vi "DAQmx Write (Raw 1D U32).vi"(0 "task/channels in":refnum<k21>, 1 "auto start":bool, 7 "data":u32[](array[numeric]), 9 "timeout":dbl=10.0 format="%0.2f", 11 "error in":errorcluster) -> (4 "task out":refnum<k21>, 10 "number of samples written per channel":u32, 15 "error out":errorcluster)   [LabVIEW 2022 SP3]
doc: "Writes multiple raw, 32-bit unsigned integer samples to a task. Use this instance for devices that use 32-bit unsigned integers as the internal representation of a sample."
uses:
  nilvaiu.dll
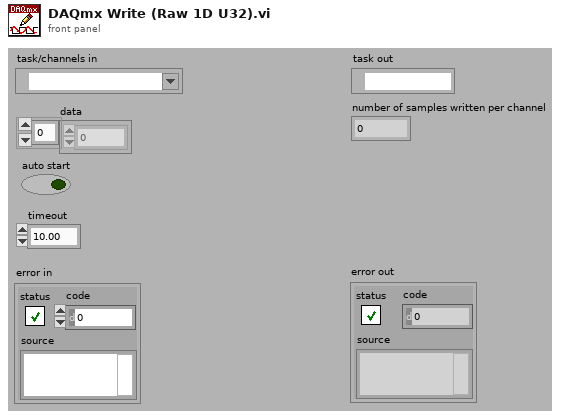
[diagram p1: front panel]
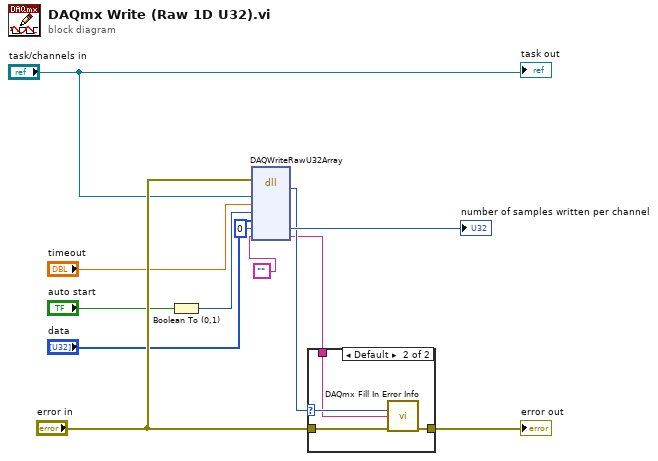
[diagram p0: block diagram]
diagram:
  n1 = Boolean To (0,1)(Boolean="auto start") -> (0, 1=w4:i16)
  n2 = dll-call lib="nilvaiu.*" fn="DAQWriteRawU32Array"(error in="error in", "taskID"="task/channels in", "timeout"="timeout", "autoStart"=w4, "data"="data", "numSamplesWriten"=u32 0, "extendedErrorInfo"="") -> ("return type"=w5:u32, "numSamplesWriten"=→"number of samples written per channel":u32, "extendedErrorInfo"=w2:string)  [unwired: 4 in, 4 out]
  n3 = case shown="Default" w5 {
    selector: w5 -> [_ w15]
    tunnel: "error in" -> [w13 w17]
    tunnel: [w13 w16] -> w12
    tunnel: w2 -> [_ w14]
    frame 0 {
    }
    frame Default {
      n4 = call "DAQmx Fill In Error Info.vi"("status code"=w15, "extended error info"=w14, "error in"=w17) -> ("error out"=w16:errorcluster)  [unwired: 1 in, 11 out]
    }
  }
  "error out" <- w12
  "task out" <- "task/channels in"
